vi "Kstar解析.vi"(11 "读取缓冲区":string) -> (3 "Status":T1)   [LabVIEW 2016, in "环境动力监测库.lvlib" / "UPS库.lvlib"]
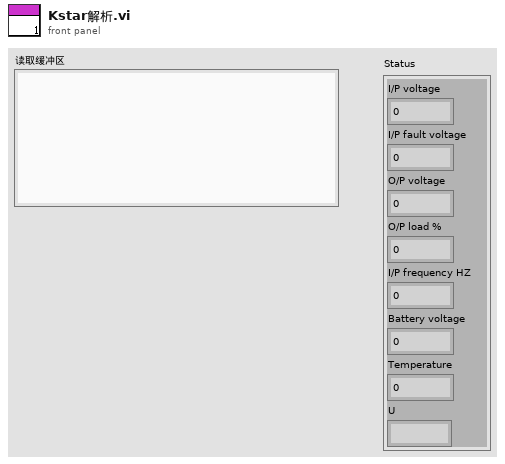
[diagram p1: front panel]
types:
  T1 = cluster{"I/P voltage":dbl, "I/P fault voltage":dbl, "O/P voltage":dbl, "O/P load %":dbl, "I/P frequency HZ":dbl, "Battery voltage":dbl, "Temperature":dbl, "U":string}
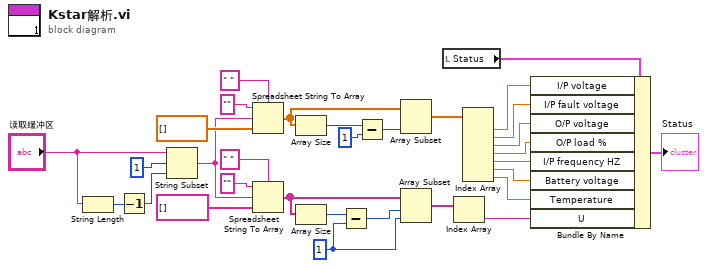
[diagram p0: block diagram]
diagram:
  w12 = 1 ("y")
  n1 = String Length(string="读取缓冲区") -> (length=w27:i32)
  n2 = Decrement(x=w27) -> (x-1=w26:i32)
  n3 = String Subset(string="读取缓冲区", offset (0)=1 ("偏移量(0)"), length (rest)=w26) -> (substring=w20:string)
  n4 = Spreadsheet String To Array(delimiter (Tab)=" " ("格式字符串"), format string="" ("格式字符串"), spreadsheet string=w20, array type (2D Dbl)=dbl[] []) -> (array=w19:dbl[])
  n5 = Spreadsheet String To Array(delimiter (Tab)=" " ("格式字符串"), format string="" ("格式字符串"), spreadsheet string=w20, array type (2D Dbl)=string[] []) -> (array=w14:string[])
  n6 = Array Size(array=w19) -> (size(s)=w18:i32)
  n7 = Array Size(array=w14) -> (size(s)=w15:i32)
  n8 = Subtract(x=w15, y=w12) -> (x-y=w13:i32)
  n9 = Subtract(x=w18, y=1) -> (x-y=w17:i32)
  n10 = Array Subset(array=w19, length=w17) -> (w11:dbl[])  [unwired: 1 in]
  n11 = Array Subset(array=w14, index=w13, length=w12) -> (w10:string[])
  n12 = local read "Status"() -> (w31:T1)
  n13 = Index Array(array=w10) -> (element=w1:string)  [unwired: 1 in]
  n14 = Index Array(array=w11) -> (element #1=w8:dbl, element #2=w7:dbl, element #3=w6:dbl, element #4=w5:dbl, element #5=w4:dbl, element #6=w3:dbl, element #7=w2:dbl)  [unwired: 7 in]
  n15 = Bundle By Name(cluster=w31, "I/P voltage"=w8, "I/P fault voltage"=w7, "O/P voltage"=w6, "O/P load %"=w5, "I/P frequency HZ"=w4, "Battery voltage"=w3, "Temperature"=w2, "U"=w1) -> (→"Status":T1)
